vi "TrafficLights_main.vi"() -> ()   [LabVIEW 2020]
uses:
  #typedef_Semofor.ctl
  #typedef_States.ctl
  #typedef_Database.ctl
  #typedef_TimerAction.ctl
panel:
  in  "STOP":bool
  out "West":T1
  out "East":T1
  out "South":T1
  out "North":T1
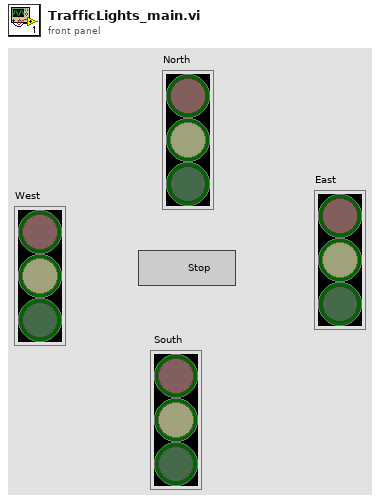
[diagram p1: front panel]
types:
  T1 = typedef "#typedef_Semofor.ctl" = cluster{"Red":bool, "Yellow":bool, "Green":bool}
  T2 = typedef "#typedef_States.ctl" = enum16{"Initialize", "Idle", "All R", "NS-R ", "NS-Y", "NS-G", "EW-R", "EW-Y", "EW-G", "All Y", "Off", "End"}
  T3 = typedef "#typedef_TimerAction.ctl" = enum16{"Reset", "TimeElapsed"}
  T4 = typedef "#typedef_Database.ctl" = cluster{"Semofory":cluster{"North":T1, " South":T1, "East":T1, "West ":T1}, "TimeToWait":cluster{"All Red":dbl, "NS G":dbl, "NS Y":dbl, "NS R":dbl, "EW G":dbl, "EW Y":dbl, "EW R":dbl, "All Y":dbl, "Off":dbl}, "Previous state":T2}
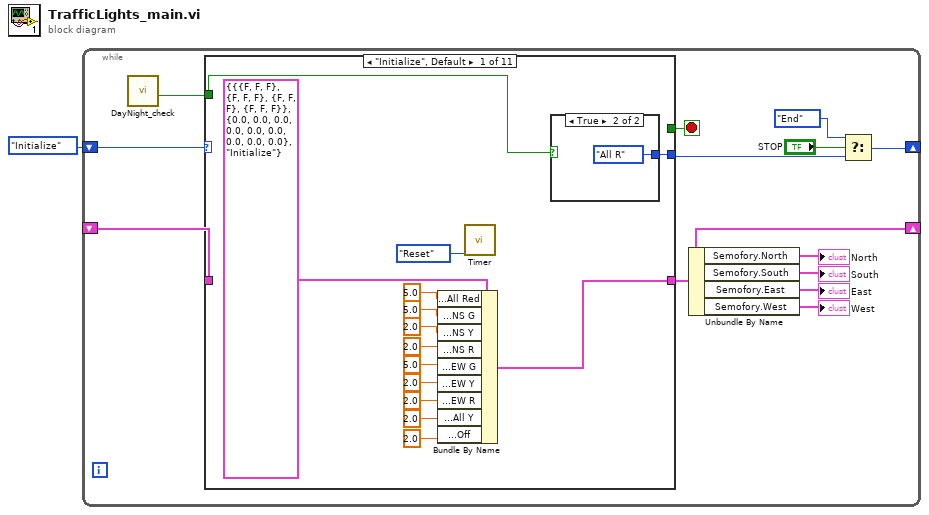
[diagram p0: block diagram]
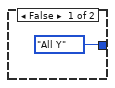
[diagram p2: hidden frame]
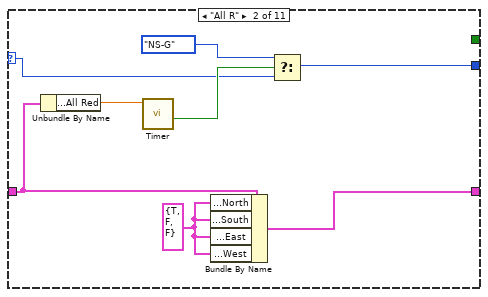
[diagram p3: hidden frame]
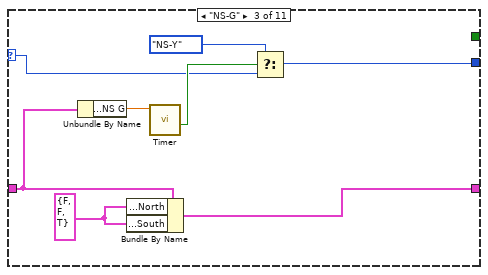
[diagram p4: hidden frame]
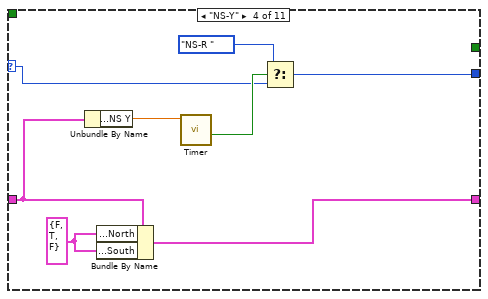
[diagram p5: hidden frame]
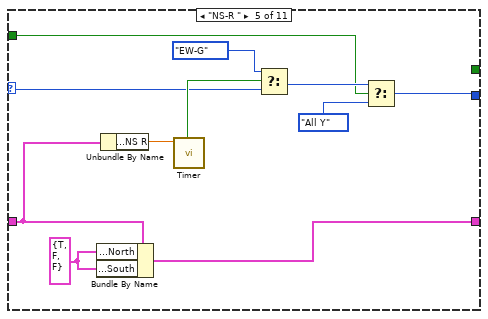
[diagram p6: hidden frame]
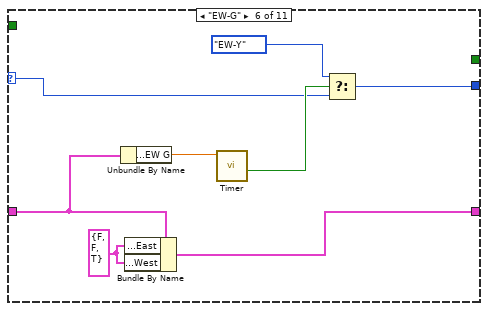
[diagram p7: hidden frame]
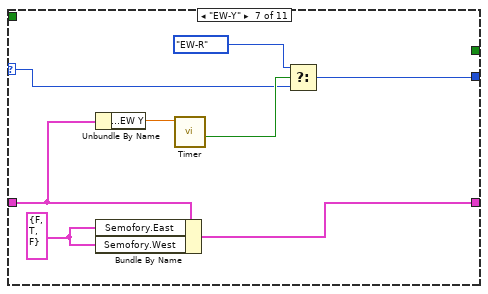
[diagram p8: hidden frame]
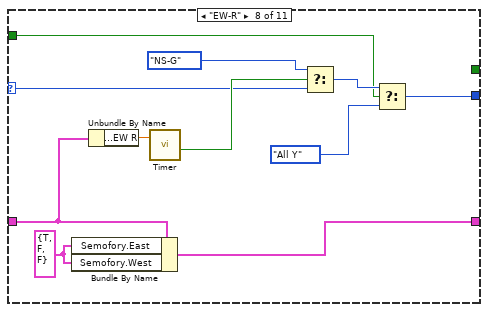
[diagram p9: hidden frame]
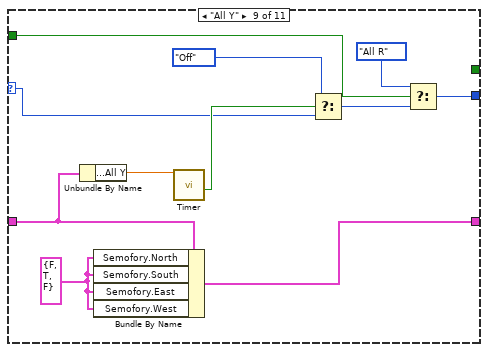
[diagram p10: hidden frame]
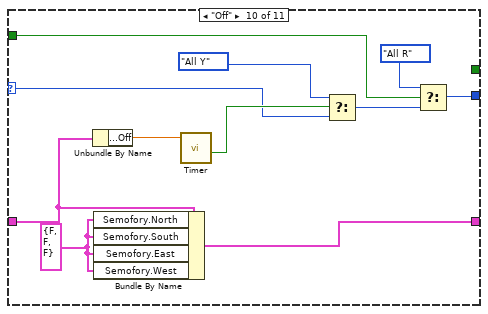
[diagram p11: hidden frame]
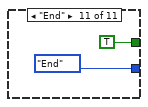
[diagram p12: hidden frame]
diagram:
  n1 = while {
    shift-right: [w13] -> _
    shift-left: _ -> [w8]
    shift-right: [w4] -> _
    shift-left: #typedef_States."Initialize" ("States") -> [w14]
    stop <- w7 stop-if-true
    n2 = call "DayNight_check.vi"() -> ("Day?"=w2:bool)  [unwired: 11 in]
    n3 = case shown="\"Initialize\", Default" w14 {
      selector: w14 -> [_ w33 w41 w47 w60 w67 w75 w87 w100 w111 _]
      tunnel: [w25 w38 w45 w53 w64 w73 w81 w92 w99 w110 _] -> w13
      tunnel: [w28 w34 w40 w49 w56 w68 w76 w82 w96 w104 #typedef_States."End" ("States")] -> w5
      tunnel: w8 -> [_ w32 w39 w48 w59 w66 w74 w86 w98 w109 _]
      tunnel: [_ _ _ _ _ _ _ _ _ _ TRUE] -> w7
      tunnel: w2 -> [w15 _ _ _ w55 _ _ w84 w95 w106 _]
      frame "Initialize", Default {
        n4 = Bundle By Name(cluster=T4 {"Semofory"={"North"={"Red"=FALSE, "Yellow"=FALSE, "Green"=FALSE}, " South"={"Red"=FALSE, "Yellow"=FALSE, "Green"=FALSE}, "East"={"Red"=FALSE, "Yellow"=FALSE, "Green"=FALSE}, "West "={"Red"=FALSE, "Yellow"=FALSE, "Green"=FALSE}}, "TimeToWait"={"All Red"=0.0, "NS G"=0.0, "NS Y"=0.0, "NS R"=0.0, "EW G"=0.0, "EW Y"=0.0, "EW R"=0.0, "All Y"=0.0, "Off"=0.0}, "Previous state"=enum."Initialize"} ("Database"), "TimeToWait.All Red"=5.0, "TimeToWait.NS G"=5.0, "TimeToWait.NS Y"=2.0, "TimeToWait.NS R"=2.0, "TimeToWait.EW G"=5.0, "TimeToWait.EW Y"=2.0, "TimeToWait.EW R"=2.0, "TimeToWait.All Y"=2.0, "TimeToWait.Off"=2.0) -> (w25:T4)
        n5 = call "Timer.vi"("Action"=#typedef_TimerAction."Reset") -> ()  [unwired: 9 in, 2 out]
        n6 = case shown="True" w15 {
          tunnel: [#typedef_States."All Y" ("States") #typedef_States."All R" ("States")] -> w28
          frame False {
          }
          frame True {
          }
        }
      }
      frame "All R" {
        w37 = T1 {"Red"=TRUE, "Yellow"=FALSE, "Green"=FALSE} ("Semofory.North")
        n7 = Unbundle By Name(w32) -> ("TimeToWait.All Red"=w31:dbl)
        n8 = call "Timer.vi"("Limit"=w31) -> ("Over limit?"=w36:bool)  [unwired: 9 in, 1 out]
        n9 = Bundle By Name(cluster=w32, "Semofory.North"=w37, "Semofory.South"=w37, "Semofory.East"=w37, "Semofory.West"=w37) -> (w38:T4)
        n10 = Select(t=#typedef_States."NS-G" ("States"), s=w36, f=w33) -> (s? t:f=w34:T2)
      }
      frame "NS-G" {
        w46 = T1 {"Red"=FALSE, "Yellow"=FALSE, "Green"=TRUE} ("Semofory.North")
        n11 = Unbundle By Name(w39) -> ("TimeToWait.NS G"=w43:dbl)
        n12 = Bundle By Name(cluster=w39, "Semofory.North"=w46, "Semofory.South"=w46) -> (w45:T4)
        n13 = call "Timer.vi"("Limit"=w43) -> ("Over limit?"=w44:bool)  [unwired: 9 in, 1 out]
        n14 = Select(t=#typedef_States."NS-Y" ("States"), s=w44, f=w41) -> (s? t:f=w40:T2)
      }
      frame "NS-Y" {
        w54 = T1 {"Red"=FALSE, "Yellow"=TRUE, "Green"=FALSE} ("Semofory.North")
        n15 = Unbundle By Name(w48) -> ("TimeToWait.NS Y"=w51:dbl)
        n16 = Bundle By Name(cluster=w48, "Semofory.North"=w54, "Semofory.South"=w54) -> (w53:T4)
        n17 = call "Timer.vi"("Limit"=w51) -> ("Over limit?"=w52:bool)  [unwired: 9 in, 1 out]
        n18 = Select(t=#typedef_States."NS-R " ("States"), s=w52, f=w47) -> (s? t:f=w49:T2)
      }
      frame "NS-R " {
        w65 = T1 {"Red"=TRUE, "Yellow"=FALSE, "Green"=FALSE} ("Semofory.North")
        n19 = Bundle By Name(cluster=w59, "Semofory.North"=w65, "Semofory.South"=w65) -> (w64:T4)
        n20 = Unbundle By Name(w59) -> ("TimeToWait.NS R"=w62:dbl)
        n21 = call "Timer.vi"("Limit"=w62) -> ("Over limit?"=w63:bool)  [unwired: 9 in, 1 out]
        n22 = Select(t=#typedef_States."EW-G" ("States"), s=w63, f=w60) -> (s? t:f=w57:T2)
        n23 = Select(t=w57, s=w55, f=#typedef_States."All Y" ("States")) -> (s? t:f=w56:T2)
      }
      frame "EW-G" {
        w72 = T1 {"Red"=FALSE, "Yellow"=FALSE, "Green"=TRUE} ("Semofory.North")
        n24 = Unbundle By Name(w66) -> ("TimeToWait.EW G"=w70:dbl)
        n25 = Bundle By Name(cluster=w66, "Semofory.East"=w72, "Semofory.West"=w72) -> (w73:T4)
        n26 = call "Timer.vi"("Limit"=w70) -> ("Over limit?"=w71:bool)  [unwired: 9 in, 1 out]
        n27 = Select(t=#typedef_States."EW-Y" ("States"), s=w71, f=w67) -> (s? t:f=w68:T2)
      }
      frame "EW-Y" {
        w80 = T1 {"Red"=FALSE, "Yellow"=TRUE, "Green"=FALSE} ("Semofory.North")
        n28 = Unbundle By Name(w74) -> ("TimeToWait.EW Y"=w78:dbl)
        n29 = Bundle By Name(cluster=w74, "Semofory.East"=w80, "Semofory.West"=w80) -> (w81:T4)
        n30 = call "Timer.vi"("Limit"=w78) -> ("Over limit?"=w79:bool)  [unwired: 9 in, 1 out]
        n31 = Select(t=#typedef_States."EW-R" ("States"), s=w79, f=w75) -> (s? t:f=w76:T2)
      }
      frame "EW-R" {
        w91 = T1 {"Red"=TRUE, "Yellow"=FALSE, "Green"=FALSE} ("Semofory.North")
        n32 = Bundle By Name(cluster=w86, "Semofory.East"=w91, "Semofory.West"=w91) -> (w92:T4)
        n33 = Unbundle By Name(w86) -> ("TimeToWait.EW R"=w89:dbl)
        n34 = call "Timer.vi"("Limit"=w89) -> ("Over limit?"=w90:bool)  [unwired: 9 in, 1 out]
        n35 = Select(t=#typedef_States."NS-G" ("States"), s=w90, f=w87) -> (s? t:f=w85:T2)
        n36 = Select(t=w85, s=w84, f=#typedef_States."All Y" ("States")) -> (s? t:f=w82:T2)
      }
      frame "All Y" {
        w97 = T1 {"Red"=FALSE, "Yellow"=TRUE, "Green"=FALSE} ("Semofory.North")
        n37 = Unbundle By Name(w98) -> ("TimeToWait.All Y"=w102:dbl)
        n38 = Bundle By Name(cluster=w98, "Semofory.North"=w97, "Semofory.South"=w97, "Semofory.East"=w97, "Semofory.West"=w97) -> (w99:T4)
        n39 = call "Timer.vi"("Limit"=w102) -> ("Over limit?"=w103:bool)  [unwired: 9 in, 1 out]
        n40 = Select(t=#typedef_States."Off" ("States"), s=w103, f=w100) -> (s? t:f=w94:T2)
        n41 = Select(t=#typedef_States."All R" ("States"), s=w95, f=w94) -> (s? t:f=w96:T2)
      }
      frame "Off" {
        w108 = T1 {"Red"=FALSE, "Yellow"=FALSE, "Green"=FALSE} ("Semofory.North")
        n42 = Unbundle By Name(w109) -> ("TimeToWait.Off"=w113:dbl)
        n43 = Bundle By Name(cluster=w109, "Semofory.North"=w108, "Semofory.South"=w108, "Semofory.East"=w108, "Semofory.West"=w108) -> (w110:T4)
        n44 = call "Timer.vi"("Limit"=w113) -> ("Over limit?"=w114:bool)  [unwired: 9 in, 1 out]
        n45 = Select(t=#typedef_States."All Y" ("States"), s=w114, f=w111) -> (s? t:f=w105:T2)
        n46 = Select(t=#typedef_States."All R" ("States"), s=w106, f=w105) -> (s? t:f=w104:T2)
      }
      frame "End" {
      }
    }
    n47 = Unbundle By Name(w13) -> ("Semofory.North"=→"North":T1, "Semofory.South"=→"South":T1, "Semofory.East"=→"East":T1, "Semofory.West"=→"West":T1)
    n48 = Select(t=#typedef_States."End" ("States"), s="STOP", f=w5) -> (s? t:f=w4:T2)
  }
